vi "Lab2_TempAvg.vi"() -> ()   [LabVIEW 2022 SP3]
uses:
  <vilib>/DAQmx/read.llb/DAQmx Read (Analog DBL 1Chan 1Samp).vi
  <vilib>/DAQmx/miscellaneous.llb/DAQmx Fill In Error Info.vi
panel:
  out "error constant":errorcluster
  in  "N [for]":i32
  out "Waveform Chart":cluster{dbl, dbl}[](graph)
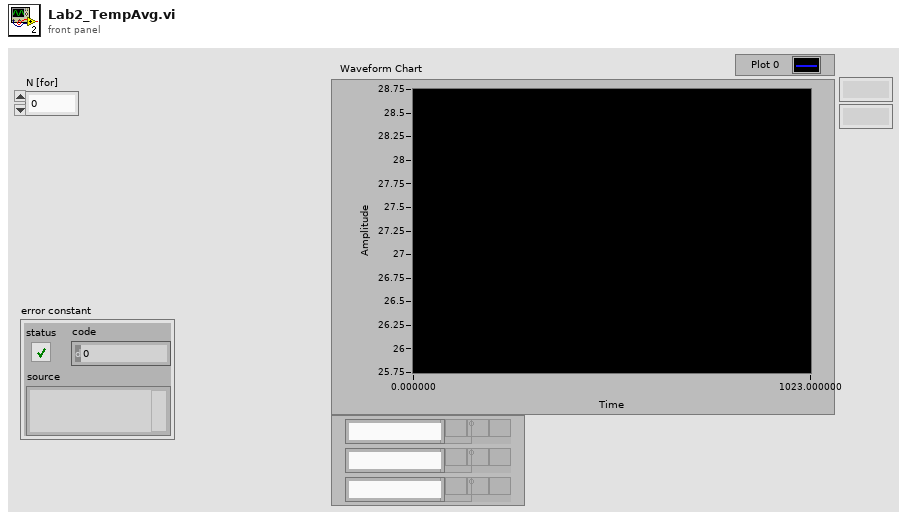
[diagram p1: front panel]
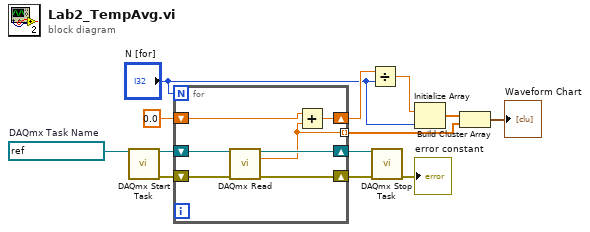
[diagram p0: block diagram]
diagram:
  w9 = refnum<k21> "Temp Sensor"  # DAQmx Task Name
  n1 = call <vilib>:"DAQmx Start Task.vi"("task/channels in"=w9) -> ("task out"=w11:refnum<k21>, "error out"=w13:errorcluster)  [unwired: 13 in]
  n2 = for {
    N: "N [for]" -> [_]
    shift-right: [w19] -> w12
    shift-left: w13 -> [w20]
    shift-right: [w17] -> w10
    shift-left: w11 -> [w18]
    shift-right: [w15] -> w5
    shift-left: 0.0 -> [w16]
    tunnel: [w14] -> w1 mode=indexing
    n3 = call-poly <vilib>:"DAQmx Read.vi"("task/channels in"=w18, "error in"=w20) -> ("task out"=w17:refnum<k21>, "data"=w14:dbl, "error out"=w19:errorcluster)  [unwired: 11 in]
    n4 = Add(x=w16, y=w14) -> (x+y=w15:dbl)
  }
  n5 = Divide(x=w5, y="N [for]") -> (x/y=w8:dbl)
  n6 = call <vilib>:"DAQmx Stop Task.vi"("task/channels in"=w10, "error in"=w12) -> ("error out"=→"error constant":errorcluster)  [unwired: 12 in, 1 out]
  n7 = Initialize Array(w8, "N [for]") -> (w7:dbl[])
  n8 = Build Cluster Array(w7, w1) -> (→"Waveform Chart":cluster{dbl, "data":dbl}[])
